vi "Car-servo-poc.vi"() -> ()   [LabVIEW 2026]
uses:
  CTI-Grove/Examples/Sourcecode/cti-drivers-lv-visa-simple/Examples/Driver/CTIPicoVISA.lvlib
panel:
  out "x*y":sgl
  in  "GPIO":i32=13
  in  "Angle":sgl(slide) scale=30.0..150.0
  out "Identity":T1
  in  "stop":bool
  in  "VISA resource name in":refnum<visa-resource-name>="ASRL1::INSTR"
  out "error out":errorcluster
  # "https://wiki.seeedstudio.com/Grove-Passive-Buzzer/"
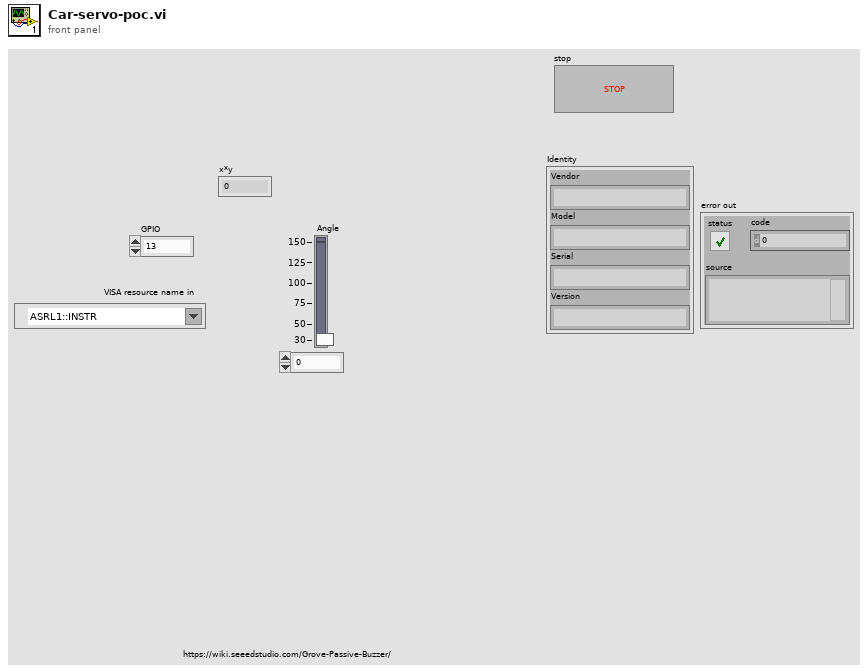
[diagram p1: front panel]
types:
  T1 = cluster{"Vendor":string, "Model":string, "Serial":string, "Version":string}
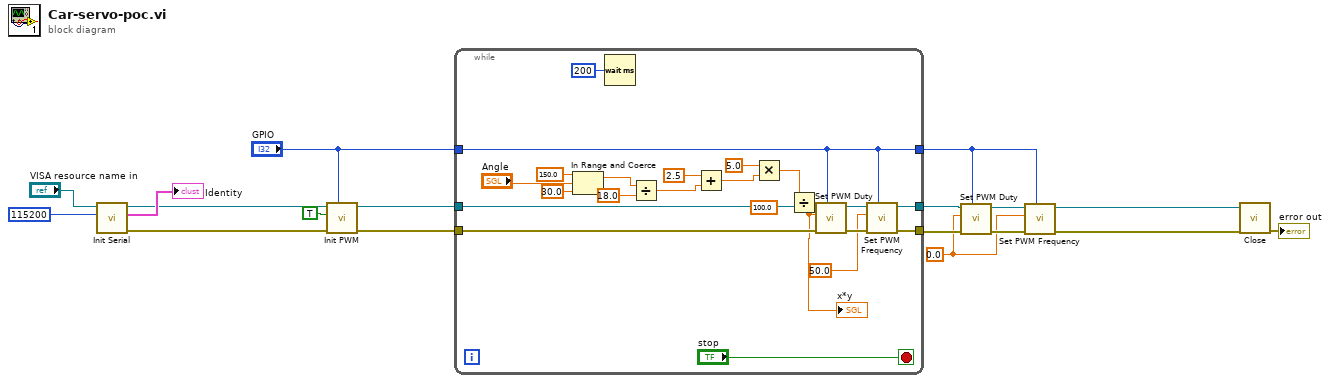
[diagram p0: block diagram]
diagram:
  w1 = sgl 0.0 ("Duty % (0-1)")
  n1 = call "Init Serial.vi"("Baud (115200)"=u32 115200, "VISA resource name in"="VISA resource name in") -> ("error out"=w13:errorcluster, "Identity"=→"Identity":T1, "VISA resource name Out"=w14:refnum<visa-resource-name>)  [unwired: 7 in]
  n2 = call "Init PWM.vi"("GPIO"="GPIO", "error in (no error)"=w13, "Enable (F)"=TRUE, "VISA resource name in"=w14) -> ("error out"=w10:errorcluster, "VISA resource name"=w3:refnum<visa-resource-name>)  [unwired: 6 in]
  n3 = while {
    tunnel: w3 -> [w36]
    tunnel: "GPIO" -> [w33]
    tunnel: w10 -> [w38]
    tunnel: [w34] -> w6
    tunnel: [w31] -> w7
    tunnel: [w33] -> w5
    stop <- "stop" stop-if-true
    n4 = In Range and Coerce(upper limit=sgl 150.0, x="Angle", lower limit=sgl 30.0) -> (coerced(x)=w27:sgl)  [unwired: 1 out]
    n5 = Wait (ms)(milliseconds to wait=u32 200) -> ()  [unwired: 1 out]
    n6 = Divide(x=w27, y=sgl 18.0) -> (x/y=w25:sgl)
    n7 = Add(x=sgl 2.5, y=w25) -> (x+y=w23:sgl)
    n8 = Multiply(x=sgl 5.0, y=w23) -> (x*y=w21:sgl)
    n9 = Divide(x=w21, y=sgl 100.0) -> (x/y=w20:sgl)
    "x*y" <- w20
    n10 = call "Set PWM Duty.vi"("GPIO"=w33, "error in (no error)"=w38, "Duty % (0-1)"=w20, "VISA resource name in"=w36) -> ("error out"=w37:errorcluster, "VISA resource name"=w35:refnum<visa-resource-name>)  [unwired: 6 in]
    n11 = call "Set PWM Frequency.vi"("GPIO"=w33, "error in (no error)"=w37, "Freq Hz"=sgl 50.0, "VISA resource name in"=w35) -> ("error out"=w34:errorcluster, "VISA resource name"=w31:refnum<visa-resource-name>)  [unwired: 6 in]
  }
  n12 = call "Set PWM Duty.vi"("GPIO"=w5, "error in (no error)"=w6, "Duty % (0-1)"=w1, "VISA resource name in"=w7) -> ("error out"=w9:errorcluster, "VISA resource name"=w8:refnum<visa-resource-name>)  [unwired: 6 in]
  n13 = call "Set PWM Frequency.vi"("GPIO"=w5, "error in (no error)"=w9, "Freq Hz"=w1, "VISA resource name in"=w8) -> ("error out"=w4:errorcluster, "VISA resource name"=w2:refnum<visa-resource-name>)  [unwired: 6 in]
  n14 = call "Close.vi"("error in (no error)"=w4, "VISA resource name in"=w2) -> ("error out"=→"error out":errorcluster)  [unwired: 9 in]
